vi "Self-Sort.vi"(7 "SubComponent List":refnum<class "1553 SubComponent.lvclass">[](array[class]), 8 "error in (no error)":errorcluster, 11 "1553 SubComponent in":refnum<class "1553 SubComponent.lvclass">) -> (0 "error out":errorcluster, 5 "SubComponent List out":refnum<class "1553 SubComponent.lvclass">[](array[class]))   [LabVIEW 2016, in "BCI-1553 API.lvlib" / "1553 SubComponent.lvclass"]
doc: "<DO NOT CALL>\n\nVirtual: All the children who decide to implement this will need to provide a means for locating themselves in the SubComonent List and updating their location appropriately."
uses:
  1553 SubComponent.lvclass
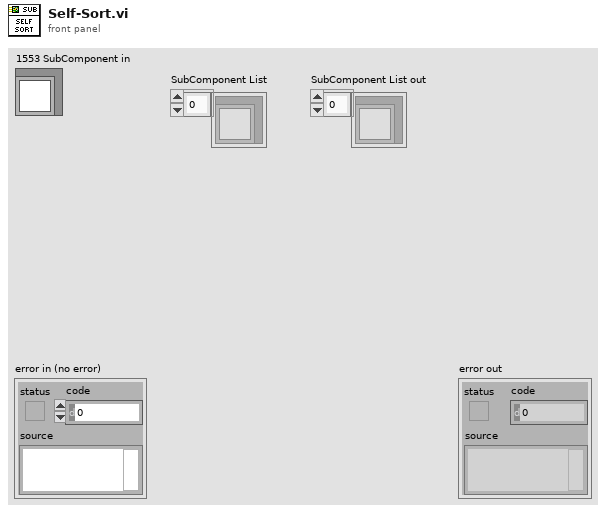
[diagram p1: front panel]
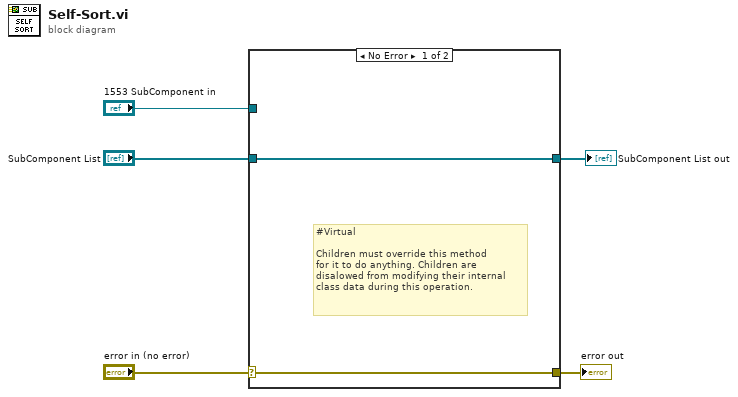
[diagram p0: block diagram]
diagram:
  n1 = case shown="No Error" "error in (no error)" {
    selector: "error in (no error)" -> [w7 w9]
    tunnel: [w7 w9] -> w4
    tunnel: "1553 SubComponent in" -> [_ _]
    tunnel: [w6 w8] -> w2
    tunnel: "SubComponent List" -> [w6 w8]
    frame No Error {
      # "#Virtual\n\nChildren must override this method\nfor it to do anything. Children are\ndisalowed from modifying their internal\nclass data during this operation."
    }
    frame Error {
    }
  }
  "error out" <- w4
  "SubComponent List out" <- w2
